vi "RotateTest.vi"() -> ()   [LabVIEW 2018]
panel:
  out "坐标输出":i32[](array[numeric])
  in  "关机":bool
  in  "近场相机":bool
  in  "偏振仪":bool
  in  "能量计":bool
  in  "功率计":bool
  out "初始化成功？":bool
  out "通信成功？":bool
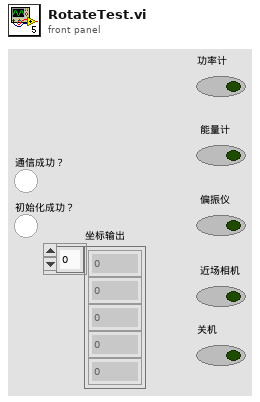
[diagram p1: front panel]
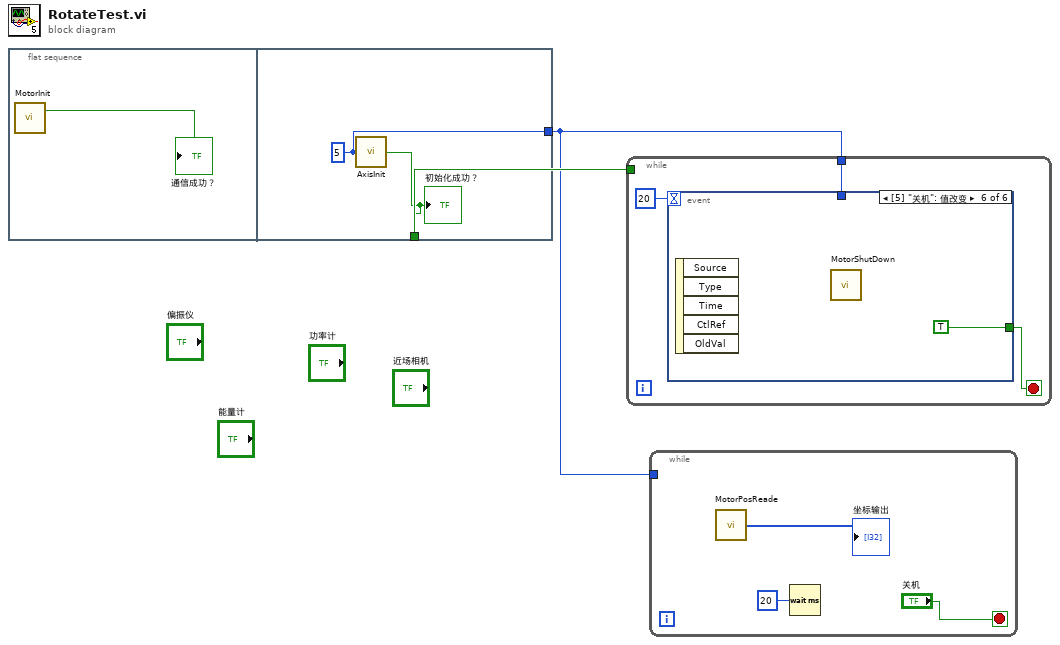
[diagram p0: block diagram]
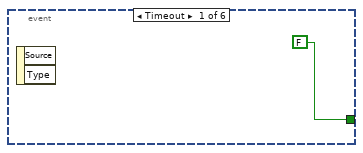
[diagram p2: hidden frame]
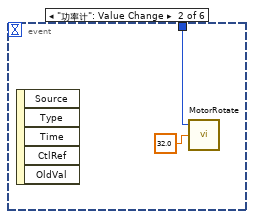
[diagram p3: hidden frame]
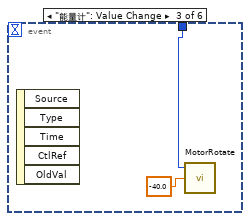
[diagram p4: hidden frame]
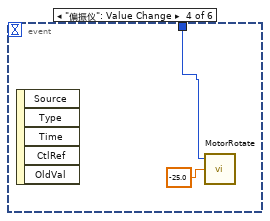
[diagram p5: hidden frame]
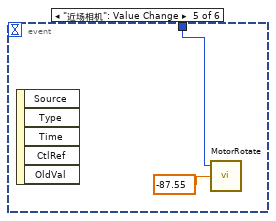
[diagram p6: hidden frame]
diagram:
  n1 = flat-sequence {
    tunnel: [w5] -> w2
    tunnel: [w4] -> w1
    frame #0 {
      n2 = call "MotorInit.vi"() -> ("通信成功？"=→"通信成功？":bool)  [unwired: 2 in, 1 out]
    }
    frame #1 {
      w4 = 5 ("axis")
      n3 = call "AxisInit.vi"("axis"=w4) -> ("初始化成功成功？"=w5:bool)
      "初始化成功？" <- w5
    }
  }
  n4 = while {
    tunnel: [w9] -> _
    tunnel: w2 -> [w9]
    tunnel: w1 -> [w8]
    stop <- w6 stop-if-true
    n5 = event shown="[5] \"关机\": 值改变" {
      selector: _ -> [_ _ _ _ _ _]
      dyn-events: _ -> [_ _ _ _ _ _]
      timeout: 20 -> [_ _ _ _ _ _]
      tunnel: w8 -> [_ w12 w13 w15 w17 _]
      tunnel: [FALSE _ _ _ _ TRUE] -> w6
      event Timeout {
        n6 = event-data() -> ()  [unwired: 1 in, 2 out]
      }
      event "功率计": Value Change {
        n7 = event-data() -> ()  [unwired: 1 in, 5 out]
        n8 = call "MotorRotate.vi"("位置"=32.0 ("角度"), "控制电机"=w12) -> ()  [unwired: 2 in, 1 out]
      }
      event "能量计": Value Change {
        n9 = event-data() -> ()  [unwired: 1 in, 5 out]
        n10 = call "MotorRotate.vi"("位置"=-40.0 ("角度"), "控制电机"=w13) -> ()  [unwired: 2 in, 1 out]
      }
      event "偏振仪": Value Change {
        n11 = event-data() -> ()  [unwired: 1 in, 5 out]
        n12 = call "MotorRotate.vi"("位置"=-25.0 ("角度"), "控制电机"=w15) -> ()  [unwired: 2 in, 1 out]
      }
      event "近场相机": Value Change {
        n13 = event-data() -> ()  [unwired: 1 in, 5 out]
        n14 = call "MotorRotate.vi"("位置"=-87.55 ("角度"), "控制电机"=w17) -> ()  [unwired: 2 in, 1 out]
      }
      event "关机": Value Change {
        n15 = event-data() -> ()  [unwired: 1 in, 5 out]
        n16 = call "MotorShutDown.vi"() -> ()  [unwired: 11 in, 1 out]
      }
    }
  }
  n17 = while {
    tunnel: w1 -> [_]
    stop <- "关机" stop-if-true
    n18 = call "MotorPosReade.vi"() -> ("坐标输出"=→"坐标输出":i32[])  [unwired: 1 in]
    n19 = Wait (ms)(milliseconds to wait=u32 20 ("等待时间（毫秒）")) -> ()  [unwired: 1 out]
  }
